vi "getMessage.vi"(8 "error in (no error)":errorcluster, 10 "key":string="welcome", 11 "simonMessages in":refnum<class "simonMessages.lvclass">) -> (0 "error out":errorcluster, 1 "Message Cluster":T1, 3 "simonMessages out":refnum<class "simonMessages.lvclass">)   [LabVIEW 2019, in "simonMessages.lvclass"]
uses:
  simonMessages.lvclass
  simonMessages.lvclass/simonMessages.ctl
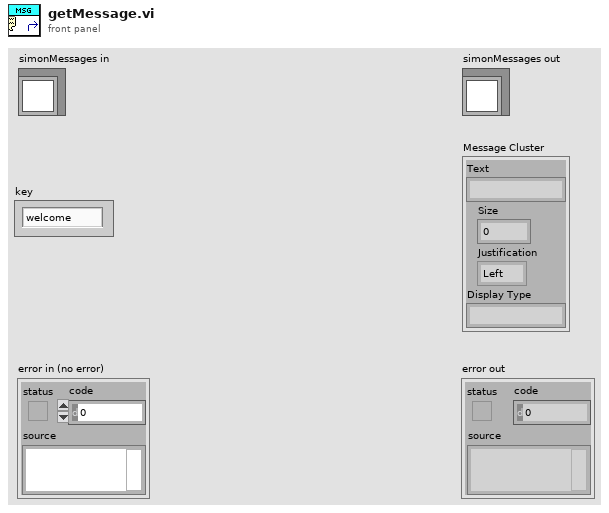
[diagram p1: front panel]
types:
  T1 = cluster{"Text":string, "Size":u8, "Justification":enum16{"Left", "Center", "Right"}, "Display Type":string}
  T2 = map{string, cluster{"Text":string, "Size":u8, "Justification":enum16{"Left", "Center", "Right"}, "Display Type":string}}
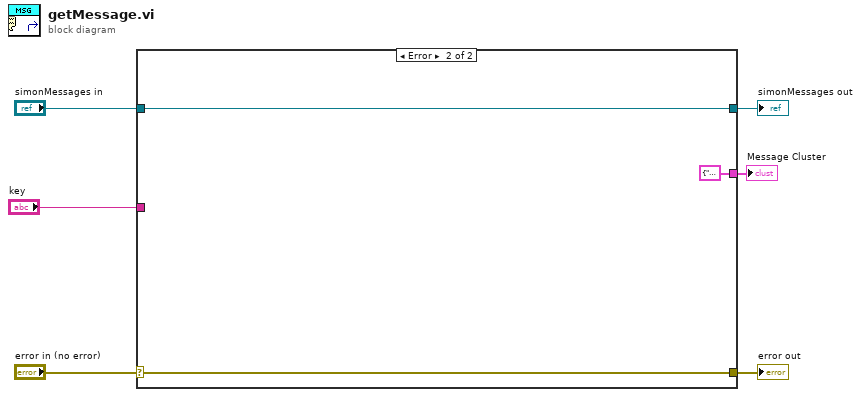
[diagram p0: block diagram]
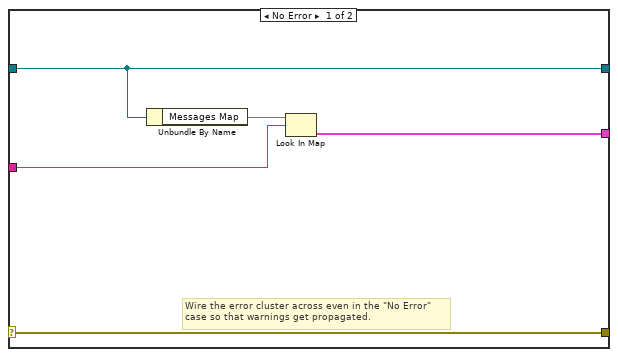
[diagram p2: hidden frame]
diagram:
  n1 = case shown="Error" "error in (no error)" {
    selector: "error in (no error)" -> [w11 w14]
    tunnel: [w11 w14] -> w5
    tunnel: [w10 w13] -> w3
    tunnel: "simonMessages in" -> [w10 w13]
    tunnel: [w8 T1 {"Text"="", "Size"=0, "Justification"=enum."Left", "Display Type"=""}] -> w1
    tunnel: "key" -> [w7 _]
    frame No Error {
      # "Wire the error cluster across even in the \"No Error\"\ncase so that warnings get propagated."
      n2 = Unbundle By Name(w10) -> ("Messages Map"=w9:T2)
      n3 = Look In Map(map=w9, key=w7) -> (value=w8:T1)  [unwired: 1 in, 1 out]
    }
    frame Error {
    }
  }
  "error out" <- w5
  "simonMessages out" <- w3
  "Message Cluster" <- w1
